vi "Scale Max Current and set AMI.vi"(8 "error in":errorcluster, 9 "CurrentToField in":refnum<class "CurrentToField.lvclass">, 10 "AMI LTS PS lvclass in":refnum<class "PS Driver AMI4xx.lvclass">, 11 "AMI HTS PS lvclass in":refnum<class "PS Driver AMI4xx.lvclass">) -> (0 "error out":errorcluster, 1 "CurrentToField out":refnum<class "CurrentToField.lvclass">, 2 "AMI LTS PS lvclass":refnum<class "PS Driver AMI4xx.lvclass">, 3 "AMI HTS PS lvclass":refnum<class "PS Driver AMI4xx.lvclass">)   [LabVIEW 2024, in "PS Driver.lvlib" / "PS Driver AMI4xx.lvclass"]
uses:
  PS Driver AMI4xx.lvclass
  CurrentToField/CurrentToField.lvclass
  CurrentToField/CurrentToField.lvclass/CurrentToField.ctl
  SCM4 Interlock/RT SubVIs/Interlock RT Globals.vi
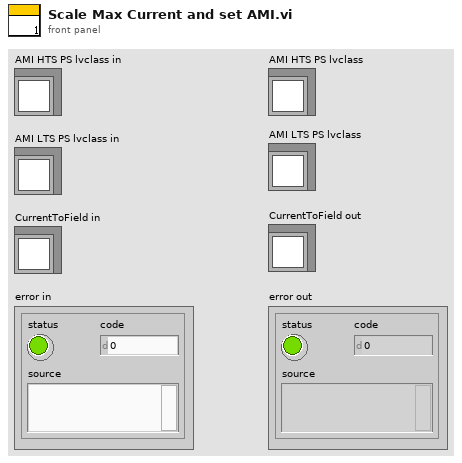
[diagram p1: front panel]
types:
  T1 = cluster{"INI key name":string, "Configuration command":string}[]
  T2 = cluster{"HTS B_I0":dbl, "LTS B_I0":dbl, "HTS Bmax":dbl, "LTS Bmax":dbl, "Max combined rate (T/min)":dbl}
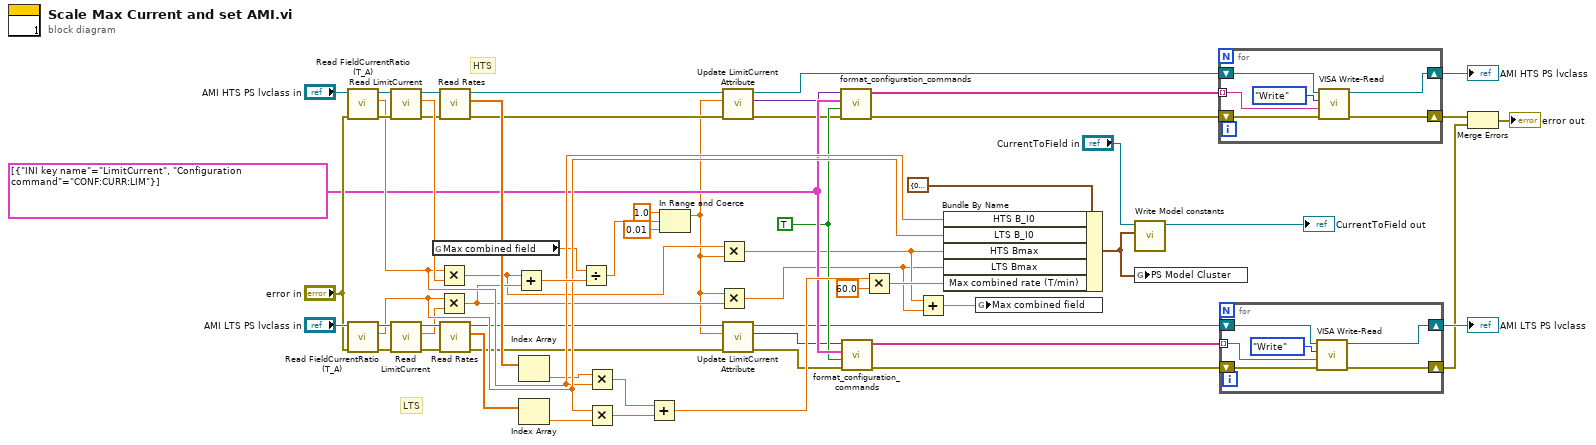
[diagram p0: block diagram]
diagram:
  w26 = TRUE ("True/false to 0/1?")
  w27 = T1 [{"INI key name"="LimitCurrent", "Configuration command"="CONF:CURR:LIM"}]
  # "LTS"
  # "HTS"
  n1 = call-dynamic "Read FieldCurrentRatio (T_A).vi"("error in (no error)"="error in", "PS Driver in"="AMI HTS PS lvclass in") -> ("error out"=w58:errorcluster, "FieldCurrentRatio (T/A)"=w44:dbl, "PS Driver out"=w59:refnum<class "PS Driver AMI4xx.lvclass">)  [unwired: 7 in]
  n2 = call-dynamic "Read FieldCurrentRatio (T_A).vi"("error in (no error)"="error in", "PS Driver in"="AMI LTS PS lvclass in") -> ("error out"=w57:errorcluster, "FieldCurrentRatio (T/A)"=w45:dbl, "PS Driver out"=w60:refnum<class "PS Driver AMI4xx.lvclass">)  [unwired: 7 in]
  n3 = call-dynamic "Read LimitCurrent.vi"("error in (no error)"=w58, "PS Driver in"=w59) -> ("error out"=w53:errorcluster, "LimitCurrent"=w56:dbl, "PS Driver out"=w54:refnum<class "PS Driver AMI4xx.lvclass">)  [unwired: 7 in]
  n4 = call-dynamic "Read LimitCurrent.vi"("error in (no error)"=w57, "PS Driver in"=w60) -> ("error out"=w52:errorcluster, "LimitCurrent"=w40:dbl, "PS Driver out"=w51:refnum<class "PS Driver AMI4xx.lvclass">)  [unwired: 7 in]
  n5 = global read "Interlock RT Globals.vi" "Max combined field"() -> (w34:dbl)
  n6 = Multiply(x=w44, y=w56) -> (x*y=w38:dbl)
  n7 = Multiply(x=w45, y=w40) -> (x*y=w39:dbl)
  n8 = call-dynamic "Read Rates.vi"("error in (no error)"=w53, "PS Driver in"=w54) -> ("error out"=w14:errorcluster, "Rates"=w42:dbl[], "PS Driver out"=w12:refnum<class "PS Driver AMI4xx.lvclass">)  [unwired: 7 in]
  n9 = call-dynamic "Read Rates.vi"("error in (no error)"=w52, "PS Driver in"=w51) -> ("error out"=w16:errorcluster, "Rates"=w41:dbl[], "PS Driver out"=w17:refnum<class "PS Driver AMI4xx.lvclass">)  [unwired: 7 in]
  n10 = Add(x=w38, y=w39) -> (x+y=w55:dbl)
  n11 = Index Array(array=w42) -> (element=w43:dbl)  [unwired: 1 in]
  n12 = Index Array(array=w41) -> (element=w28:dbl)  [unwired: 1 in]
  n13 = Divide(x=w34, y=w55) -> (x/y=w6:dbl)
  n14 = Multiply(x=w43, y=w44) -> (x*y=w49:dbl)
  n15 = Multiply(x=w45, y=w28) -> (x*y=w50:dbl)
  n16 = Add(x=w49, y=w50) -> (x+y=w48:dbl)
  n17 = In Range and Coerce(upper limit=1.0 ("x"), x=w6, lower limit=0.01) -> (coerced(x)=w4:dbl)  [unwired: 1 out]
  n18 = Multiply(x=w38, y=w4) -> (x*y=w3:dbl)
  n19 = Multiply(x=w4, y=w39) -> (x*y=w2:dbl)
  n20 = call-dynamic "Update LimitCurrent Attribute.vi"("error in"=w14, "Scale From Config Max"=w4, "PS Driver in"=w12) -> ("error out"=w13:errorcluster, "Variant"=w9:variant, "PS Driver out"=w11:refnum<class "PS Driver AMI4xx.lvclass">)  [unwired: 6 in]
  n21 = call-dynamic "Update LimitCurrent Attribute.vi"("error in"=w16, "Scale From Config Max"=w4, "PS Driver in"=w17) -> ("error out"=w15:errorcluster, "Variant"=w8:variant, "PS Driver out"=w10:refnum<class "PS Driver AMI4xx.lvclass">)  [unwired: 6 in]
  n22 = call "format_configuration_commands.vi"("error in (no error)"=w13, "True/false to 0/1?"=w26, "Configuration editables"=w27, "Config data in"=w9) -> ("error out"=w21:errorcluster, "Configuration commands"=w24:string[])  [unwired: 6 in]
  n23 = call "format_configuration_commands.vi"("error in (no error)"=w15, "True/false to 0/1?"=w26, "Configuration editables"=w27, "Config data in"=w8) -> ("error out"=w22:errorcluster, "Configuration commands"=w23:string[])  [unwired: 6 in]
  n24 = Multiply(x=w48, y=60.0) -> (x*y=w47:dbl)
  n25 = Add(x=w3, y=w2) -> (x+y=w1:dbl)
  n26 = Bundle By Name(cluster=T2 {"HTS B_I0"=0.0, "LTS B_I0"=0.0, "HTS Bmax"=0.0, "LTS Bmax"=0.0, "Max combined rate (T/min)"=0.0} ("Model constants"), "HTS B_I0"=w44, "LTS B_I0"=w45, "HTS Bmax"=w3, "LTS Bmax"=w2, "Max combined rate (T/min)"=w47) -> (w30:T2)
  n27 = global write "Interlock RT Globals.vi" "Max combined field"(w1) -> ()
  n28 = call "Write Model constants.vi"("Model constants"=w30, "CurrentToField in"="CurrentToField in") -> ("CurrentToField out"=→"CurrentToField out":refnum<class "CurrentToField.lvclass">)  [unwired: 9 in]
  n29 = global write "Interlock RT Globals.vi" "PS Model Cluster"(w30) -> ()
  n30 = for {
    shift-right: [w61] -> w19
    shift-left: w21 -> [w64]
    shift-right: [w62] -> w25
    shift-left: w11 -> [w65]
    tunnel: w24 -> [w63] mode=indexing
    n31 = call "VISA Write-Read.vi"("error in (no error)"=w64, "Command String"=w63, "Action"=enum16{"Write", "Read", "Write & Read"}."Write", "PS Driver.lvlib:PS Driver AMI4xx.lvclass"=w65) -> ("error out"=w61:errorcluster, "PS Driver.lvlib:PS Driver AMI4xx.lvclass out"=w62:refnum<class "PS Driver AMI4xx.lvclass">)  [unwired: 4 in, 2 out]
  }
  "AMI HTS PS lvclass" <- w25
  n32 = for {
    shift-right: [w67] -> w18
    shift-left: w22 -> [w70]
    shift-right: [w68] -> w20
    shift-left: w10 -> [w71]
    tunnel: w23 -> [w69] mode=indexing
    n33 = call "VISA Write-Read.vi"("error in (no error)"=w70, "Command String"=w69, "Action"=enum16{"Write", "Read", "Write & Read"}."Write", "PS Driver.lvlib:PS Driver AMI4xx.lvclass"=w71) -> ("error out"=w67:errorcluster, "PS Driver.lvlib:PS Driver AMI4xx.lvclass out"=w68:refnum<class "PS Driver AMI4xx.lvclass">)  [unwired: 4 in, 2 out]
  }
  "AMI LTS PS lvclass" <- w20
  n34 = Merge Errors(w19, w18) -> (→"error out":errorcluster)
